vi "QA-Find FP Controls.vi"(8 "error in (no error)":errorcluster, 10 "FP Controls":T1, 11 "VI Refnum":refnum<vi>) -> (0 "error out":errorcluster, 2 "FP Controls out":T1, 3 "VI Refnum out":refnum<vi>)   [LabVIEW 2015]
uses:
  QA-FP Controls.ctl
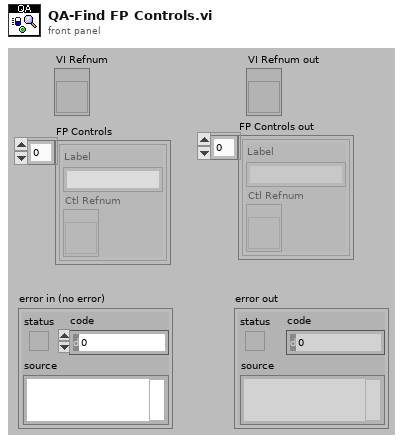
[diagram p1: front panel]
types:
  T1 = typedef "QA-FP Controls.ctl" = cluster{"Label":string, "Ctl Refnum":refnum<vi>}[]
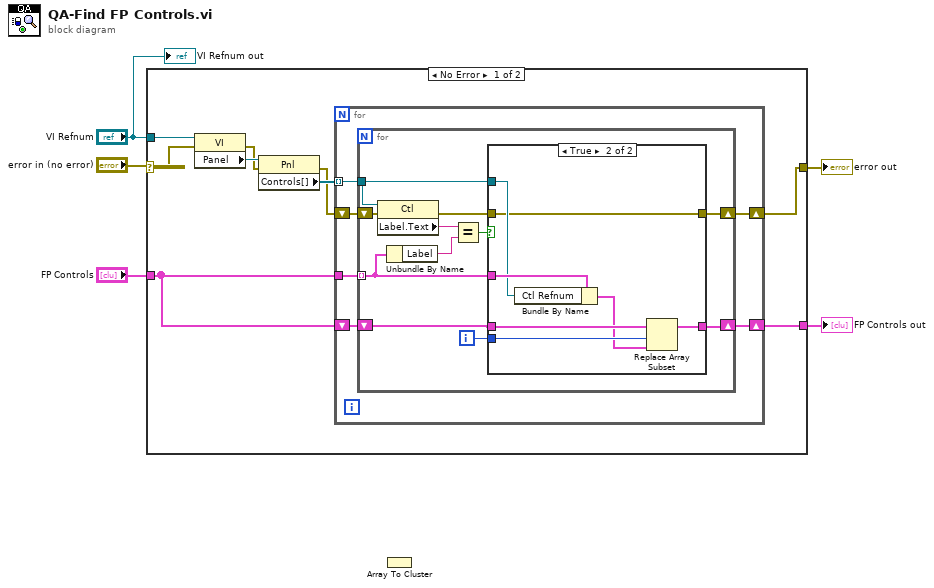
[diagram p0: block diagram]
diagram:
  n1 = case shown="No Error" "error in (no error)" {
    selector: "error in (no error)" -> [w9 w42]
    tunnel: [w14 w41] -> w5
    tunnel: "FP Controls" -> [w13 w41]
    tunnel: "VI Refnum" -> [w10 _]
    tunnel: [w7 w42] -> w2
    frame No Error {
      n2 = property class="VI"(reference=w10, error in=w9) -> (error out=w8:errorcluster, "Panel"=w11:refnum<vi>)  [unwired: 1 out]
      n3 = property class="Pnl"(reference=w11, error in=w8) -> (error out=w6:errorcluster, "Controls[]"=w12:refnum<vi>[])  [unwired: 1 out]
      n4 = for {
        tunnel: w12 -> [w20] mode=indexing
        tunnel: w13 -> [w19]
        shift-right: [w17] -> w14
        shift-left: w13 -> [w18]
        shift-right: [w16] -> w7
        shift-left: w6 -> [w15]
        n5 = for {
          tunnel: w20 -> [w31]
          tunnel: w19 -> [w25] mode=indexing
          shift-right: [w24] -> w17
          shift-left: w18 -> [w27]
          shift-right: [w21] -> w16
          shift-left: w15 -> [w23]
          i -> [w26]
          n6 = property class="Ctl"(reference=w31, error in=w23) -> (error out=w22:errorcluster, "Label.Text"=w30:string)  [unwired: 1 out]
          n7 = Unbundle By Name(w25) -> ("Label"=w28:string)
          n8 = Equal?(x=w30, y=w28) -> (x = y?=w29:bool)
          n9 = case shown="True" w29 {
            tunnel: w31 -> [_ w37]
            tunnel: w27 -> [w33 w40]
            tunnel: w26 -> [_ w39]
            tunnel: w25 -> [_ w38]
            tunnel: [w33 w35] -> w24
            tunnel: w22 -> [w32 w34]
            tunnel: [w32 w34] -> w21
            frame False {
            }
            frame True {
              n10 = Bundle By Name(cluster=w38, "Ctl Refnum"=w37) -> (w36:cluster{"Label":string, "Ctl Refnum":refnum<vi>})
              n11 = Replace Array Subset(array=w40, new element=w36, index=w39) -> (w35:T1)
            }
          }
        }
      }
    }
    frame Error {
    }
  }
  "FP Controls out" <- w5
  "error out" <- w2
  n12 = Array To Cluster() -> ()  [unwired: 1 in, 1 out]
  "VI Refnum out" <- "VI Refnum"
